vi "Temp fin.vi"() -> ()   [LabVIEW 2020]
panel:
  out "current time":timestamp
  in  "F":dbl
  in  "C":dbl
  out "F to C":dbl
  out "C to F":dbl
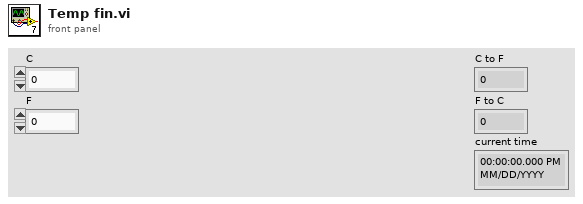
[diagram p1: front panel]
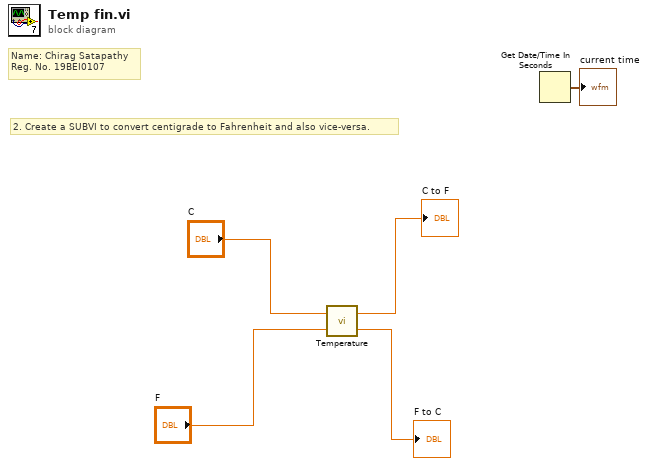
[diagram p0: block diagram]
diagram:
  # "Name: Chirag Satapathy\nReg. No. 19BEI0107"
  # "2. Create a SUBVI to convert centigrade to Fahrenheit and also vice-versa."
  n1 = call "Temperature.vi"("F"="F", "C"="C") -> ("F to C"=→"F to C":dbl, "C to F"=→"C to F":dbl)
  n2 = Get Date/Time In Seconds() -> (seconds since 1Jan1904=→"current time":timestamp)
